vi "Adjust Pod Radii.vi"(10 "Center of Rotation":cluster{"x":dbl, "y":dbl}, 11 "Radii (ft)":T1 {"Right Back Position" format="%.2f"; "Right Front Position" format="%.2f"; "Left Back Position" format="%.2f"; "Left Front Position" format="%.2f"}) -> (3 "Adjusted Radii (ft)":cluster{dbl[], dbl[], dbl[], dbl[]})   [LabVIEW 2025]
uses:
  swerve-template/Type Definitions/Data/Pod Positions.ctl
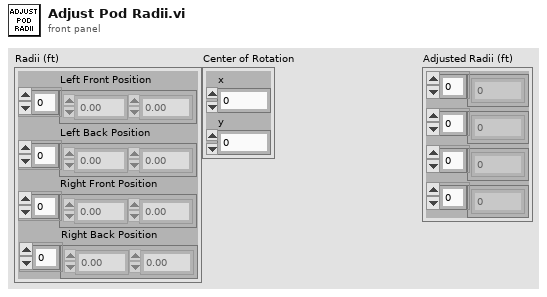
[diagram p1: front panel]
types:
  T1 = typedef "Pod Positions.ctl" = cluster{"Left Front Position":dbl[], "Left Back Position":dbl[], "Right Front Position":dbl[], "Right Back Position":dbl[]}
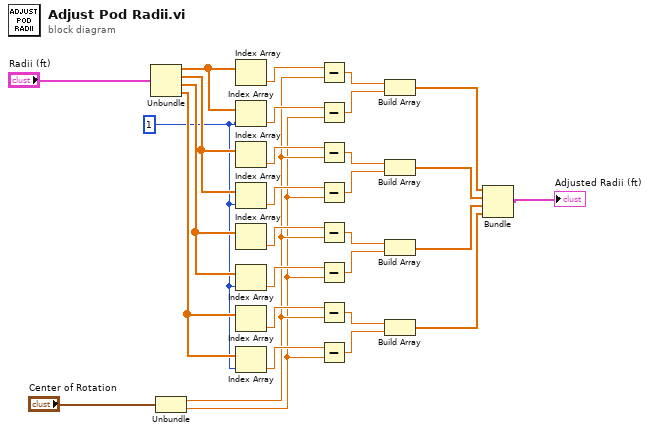
[diagram p0: block diagram]
diagram:
  w26 = 1 ("index")
  n1 = Unbundle("Radii (ft)") -> ("Left Front Position"=w27:dbl[], "Left Back Position"=w30:dbl[], "Right Front Position"=w29:dbl[], "Right Back Position"=w28:dbl[])
  n2 = Unbundle("Center of Rotation") -> ("x"=w3:dbl, "y"=w2:dbl)
  n3 = Index Array(array=w27) -> (element=w25:dbl)  [unwired: 1 in]
  n4 = Index Array(array=w27, index=w26) -> (element=w24:dbl)
  n5 = Index Array(array=w30) -> (element=w23:dbl)  [unwired: 1 in]
  n6 = Index Array(array=w30, index=w26) -> (element=w22:dbl)
  n7 = Index Array(array=w29) -> (element=w21:dbl)  [unwired: 1 in]
  n8 = Index Array(array=w29, index=w26) -> (element=w20:dbl)
  n9 = Index Array(array=w28) -> (element=w19:dbl)  [unwired: 1 in]
  n10 = Index Array(array=w28, index=w26) -> (element=w18:dbl)
  n11 = Subtract(x=w25, y=w3) -> (x-y=w17:dbl)
  n12 = Subtract(x=w24, y=w2) -> (x-y=w16:dbl)
  n13 = Subtract(x=w23, y=w3) -> (x-y=w15:dbl)
  n14 = Subtract(x=w22, y=w2) -> (x-y=w14:dbl)
  n15 = Subtract(x=w21, y=w3) -> (x-y=w13:dbl)
  n16 = Subtract(x=w20, y=w2) -> (x-y=w12:dbl)
  n17 = Subtract(x=w19, y=w3) -> (x-y=w11:dbl)
  n18 = Subtract(x=w18, y=w2) -> (x-y=w10:dbl)
  n19 = Build Array(w17, w16) -> (w9:dbl[])
  n20 = Build Array(w15, w14) -> (w8:dbl[])
  n21 = Build Array(w13, w12) -> (w7:dbl[])
  n22 = Build Array(w11, w10) -> (w6:dbl[])
  n23 = Bundle(w9, w8, w7, w6) -> (→"Adjusted Radii (ft)":cluster{dbl[], dbl[], dbl[], dbl[]})  [unwired: 1 in]
